vi "MakeYourOwn.vi"() -> ()   [LabVIEW 2022 SP3]
uses:
  _LVsubs/MakeYourOwn/Serial_Port.xctl
  _LVsubs/MakeYourOwn/Code.xctl
  _LVsubs/MakeYourOwn/File Tree.xctl
panel:
  out "good?":bool
  in  "version":bool
  in  "reconnect":bool
  in  "File Tree":path(xcontrol)
  in  "Settings":bool
  in  "Spike":bool
  in  "Tab Control":enum32{"Chart", "Scope", "Last lines"}(tab)
  out "Chart":dbl(graph)
  out "Graph":dbl[](graph)
  in  "new lines":string[](array[string])
  in  "Serial_Port":T2(xcontrol)
  out "Console":string
  in  "Path":path
  in  "Code":string(xcontrol)
  in  "Send Code":bool
  in  "CtrlE":bool
  in  "Stop":bool
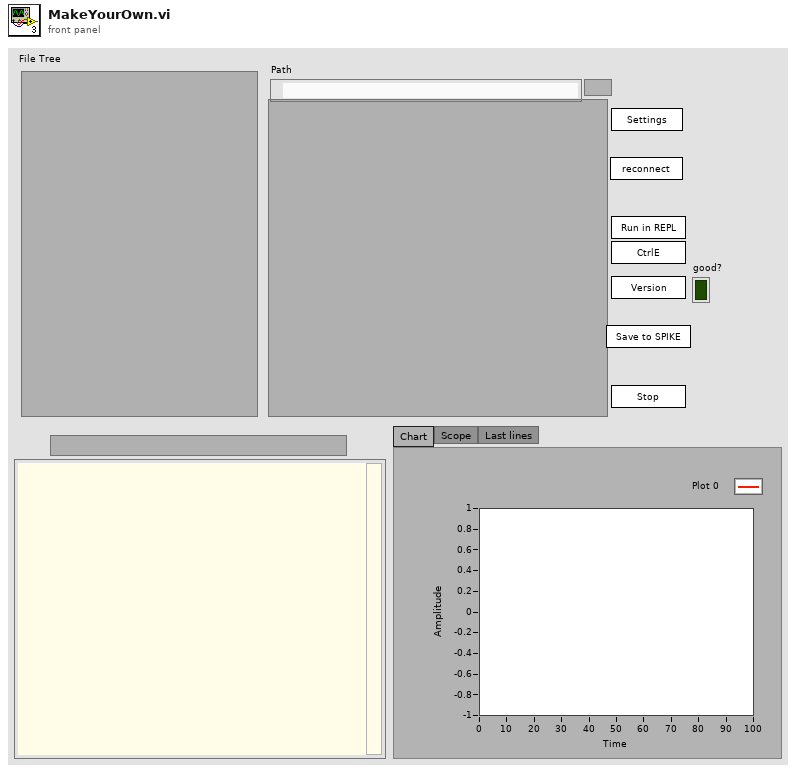
[diagram p1: front panel]
types:
  T1 = typedef "Processors.ctl" = enum16{"SPIKE", "Pi", "Pi_ssh", "OpenMV", "Dunio"}
  T2 = cluster{"session":refnum<k35>, "PyPath":path, "Processor":T1, "Port":string, "version":string}
  T3 = typedef "Preferences.ctl" = cluster{"python":string, "arduino CLI":path, "pythonCodes":cluster{"pythonCode":path, "Color":u32}[], "FontSize":u8, "Text Colors":cluster{"Quote":u32, "function":u32, "Python":u32, "Comment":u32, "Triple Quote":u32, "Text":u32}, "SSH Logins":cluster{"IP Address":string, "Username":string, "password":string}[], "packet size":u8}
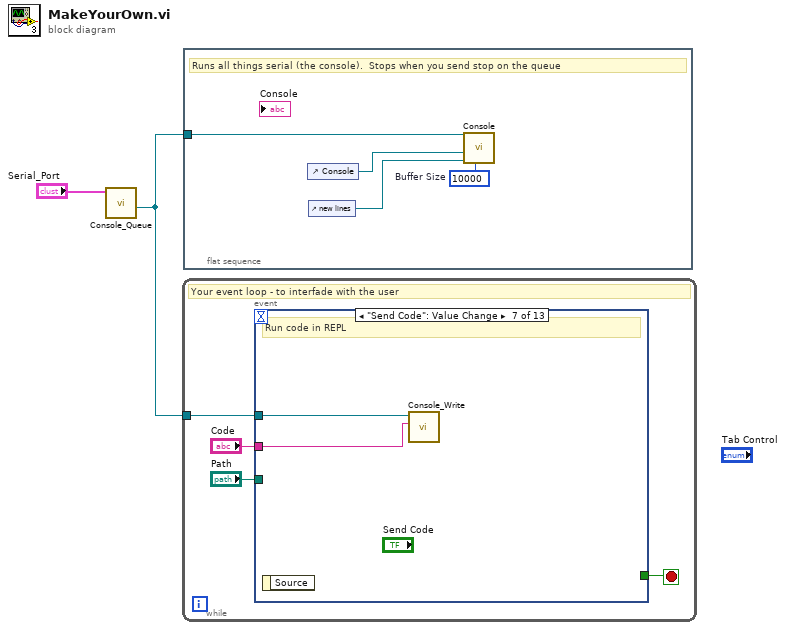
[diagram p0: block diagram]
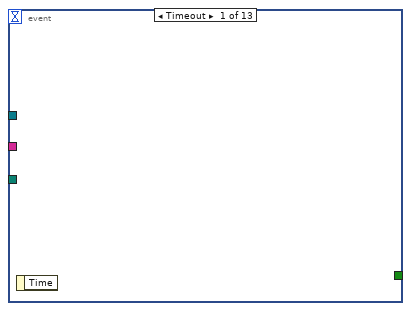
[diagram p2: hidden frame]
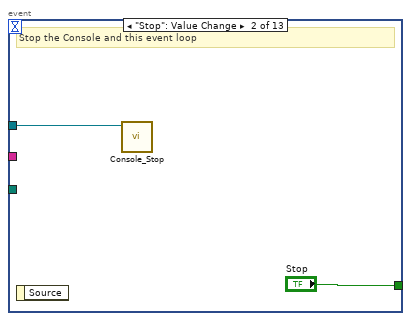
[diagram p3: hidden frame]
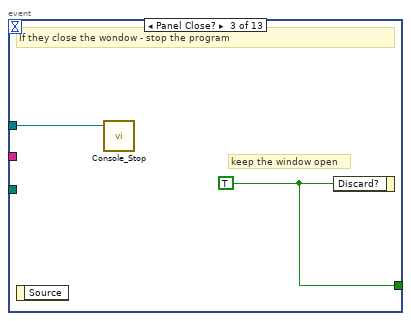
[diagram p4: hidden frame]
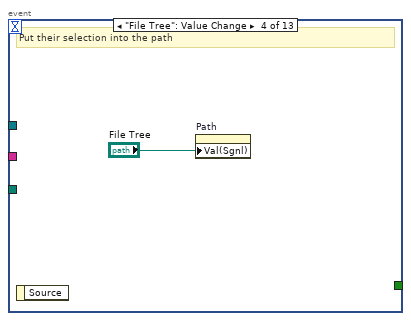
[diagram p5: hidden frame]
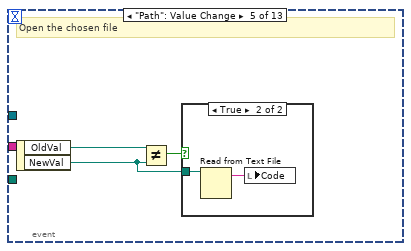
[diagram p6: hidden frame]
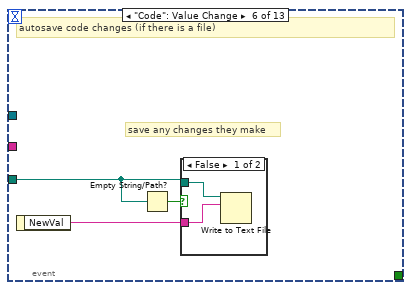
[diagram p8: hidden frame]
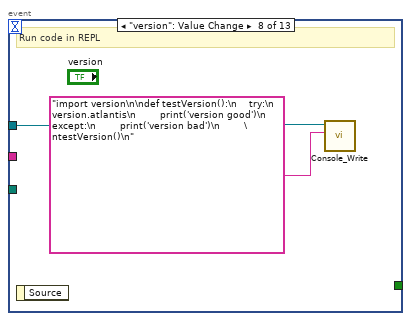
[diagram p10: hidden frame]
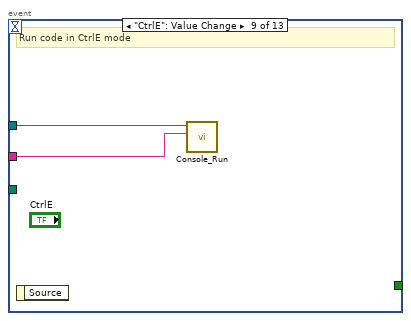
[diagram p11: hidden frame]
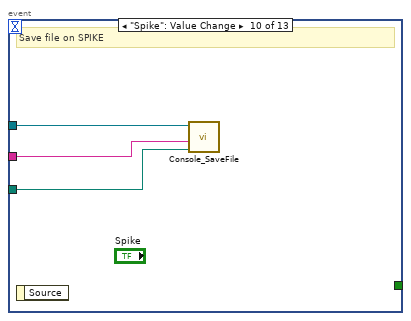
[diagram p12: hidden frame]
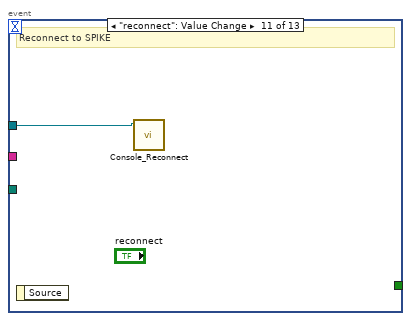
[diagram p13: hidden frame]
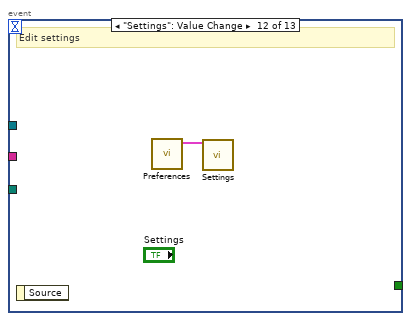
[diagram p14: hidden frame]
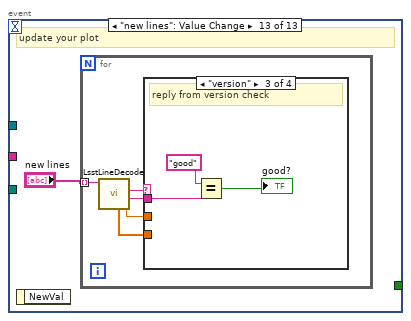
[diagram p15: hidden frame]
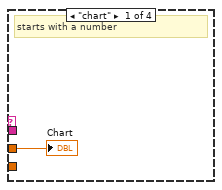
[diagram p16: hidden frame]
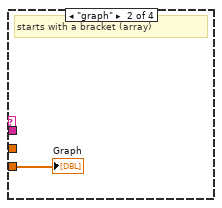
[diagram p17: hidden frame]
diagram:
  n1 = call "Console_Queue.vi"("Serial_Port"="Serial_Port") -> ("Queue out"=w2:refnum<queue>)  [unwired: 9 in, 1 out]
  n2 = while {
    tunnel: w2 -> [w5]
    stop <- w6 stop-if-true
    # "Your event loop - to interfade with the user"
    n3 = event shown="[6] \"Send Code\": Value Change" {
      selector: _ -> [_ _ _ _ _ _ _ _ _ _ _ _ _]
      dyn-events: _ -> [_ _ _ _ _ _ _ _ _ _ _ _ _]
      timeout: _ -> [_ _ _ _ _ _ _ _ _ _ _ _ _]
      tunnel: [_ "Stop" w10 _ _ _ _ _ _ _ _ _ _] -> w6
      tunnel: w5 -> [_ w7 w9 _ _ _ w23 w25 w27 w30 w31 _ _]
      tunnel: "Path" -> [_ _ _ _ _ w17 _ _ _ w28 _ _ _]
      tunnel: "Code" -> [_ _ _ _ _ _ w22 _ w26 w29 _ _ _]
      event Timeout {
        n4 = event-data() -> ()  [unwired: 1 in, 1 out]
      }
      event "Stop": Value Change {
        # "Stop the Console and this event loop"
        n5 = event-data() -> ()  [unwired: 1 in, 1 out]
        n6 = call "Console_Stop.vi"("Queue in"=w7) -> ()  [unwired: 11 in]
      }
      event Panel Close? {
        w10 = TRUE ("Discard?")
        # "keep the window open"
        # "If they close the wondow - stop the program"
        n7 = event-data() -> ()  [unwired: 1 in, 1 out]
        n8 = call "Console_Stop.vi"("Queue in"=w9) -> ()  [unwired: 11 in]
        n9 = event-data("Discard?"=w10) -> ()  [unwired: 1 in, 1 out]
      }
      event "File Tree": Value Change {
        # "Put their selection into the path"
        n10 = event-data() -> ()  [unwired: 1 in, 1 out]
        n11 = property on="Path" class="Path"("Val(Sgnl)"="File Tree") -> ()  [unwired: 2 in, 2 out]
      }
      event "Path": Value Change {
        # "Open the chosen file"
        n12 = event-data() -> ("OldVal"=w14:path, "NewVal"=w12:path)  [unwired: 1 in]
        n13 = Not Equal?(x=w14, y=w12) -> (x != y?=w13:bool)
        n14 = case shown="True" w13 {
          tunnel: w12 -> [_ w16]
          frame False {
          }
          frame True {
            n15 = Read from Text File(file (use dialog)=w16) -> (text=w15:string)  [unwired: 3 in, 3 out]
            n16 = local write "Code"(w15) -> ()
          }
        }
      }
      event "Code": Value Change {
        # "save any changes they make"
        # "autosave code changes (if there is a file)"
        n17 = event-data() -> ("NewVal"=w19:string)  [unwired: 1 in]
        n18 = Empty String/Path?(string/path=w17) -> (empty?=w18:bool)
        n19 = case shown="False" w18 {
          tunnel: w19 -> [w21 _]
          tunnel: w17 -> [w20 _]
          frame False {
            n20 = Write to Text File(file (use dialog)=w20, text=w21) -> ()  [unwired: 2 in, 3 out]
          }
          frame True {
          }
        }
      }
      event "Send Code": Value Change {
        # "Run code in REPL"
        n21 = event-data() -> ()  [unwired: 1 in, 1 out]
        n22 = call "Console_Write.vi"("Code"=w22, "Queue in"=w23) -> ()  [unwired: 10 in]
      }
      event "version": Value Change {
        # "Run code in REPL"
        n23 = event-data() -> ()  [unwired: 1 in, 1 out]
        n24 = call "Console_Write.vi"("Code"="import version\n\ndef testVersion():\n    try:\n        version.atlantis\n        print('version good')\n    except:\n        print('version bad')\n        \ntestVersion()\n", "Queue in"=w25) -> ()  [unwired: 10 in]
      }
      event "CtrlE": Value Change {
        # "Run code in CtrlE mode"
        n25 = event-data() -> ()  [unwired: 1 in, 1 out]
        n26 = call "Console_Run.vi"("Code"=w26, "Queue in"=w27) -> ()  [unwired: 10 in]
      }
      event "Spike": Value Change {
        # "Save file on SPIKE"
        n27 = event-data() -> ()  [unwired: 1 in, 1 out]
        n28 = call "Console_SaveFile.vi"("Path"=w28, "Code"=w29, "Queue in"=w30) -> ()  [unwired: 9 in]
      }
      event "reconnect": Value Change {
        # "Reconnect to SPIKE"
        n29 = event-data() -> ()  [unwired: 1 in, 1 out]
        n30 = call "Console_Reconnect.vi"("Queue in"=w31) -> ()  [unwired: 11 in]
      }
      event "Settings": Value Change {
        # "Edit settings"
        n31 = event-data() -> ()  [unwired: 1 in, 1 out]
        n32 = call "Preferences.vi"() -> ("Preferences out"=w32:T3)  [unwired: 10 in, 1 out]
        n33 = call "Settings.vi"("Prefs"=w32) -> ()  [unwired: 10 in, 1 out]
      }
      event "new lines": Value Change {
        # "update your plot"
        n34 = event-data() -> ()  [unwired: 1 in, 1 out]
        n35 = for {
          tunnel: "new lines" -> [w34] mode=indexing
          n36 = call "LsstLineDecode.vi"("new lines"=w34) -> ("Chart"=w37:dbl, "payload"=w35:string, "cmd"=w38:string, "Graph"=w36:dbl[])  [unwired: 6 in, 1 out]
          n37 = case shown="\"version\"" w38 {
            tunnel: w37 -> [w39 _ _ _]
            tunnel: w36 -> [_ w40 _ _]
            tunnel: w35 -> [_ _ w43 _]
            frame "chart" {
              # "starts with a number"
              "Chart" <- w39
            }
            frame "graph" {
              # "starts with a bracket (array)"
              "Graph" <- w40
            }
            frame "version" {
              # "reply from version check"
              n38 = Equal?(x="good", y=w43) -> (x = y?=→"good?":bool)
            }
            frame Default {
              # "Some command"
            }
          }
        }
      }
    }
  }
  n39 = flat-sequence {
    tunnel: w2 -> [w44]
    frame #0 {
      w46 = 10000  # Buffer Size
      # "Runs all things serial (the console).  Stops when you send stop on the queue"
      n40 = control-ref of="Console"() -> (w47:refnum<vi>)
      n41 = control-ref of="new lines"() -> (w45:refnum<vi>)
      n42 = call "Console.vi"("Buffer Size"=w46, "Last Lines"=w45, "Remote Console"=w47, "Queue in"=w44) -> ()  [unwired: 8 in]
    }
  }
